vi "Add User.vi"(8 "error in":errorcluster) -> (0 "error Out":errorcluster)   [LabVIEW 2022 SP3]
uses:
  <vilib>/Utility/file.llb/Read Delimited Spreadsheet (string).vi
  <vilib>/Utility/file.llb/Write Delimited Spreadsheet (string).vi
panel:
  in  "EXIT":bool
  out "Decoded Data":string[][](array[string])
  in  "ACCESS LEVEL":string(combo)
  in  "Add User":bool
  in  "ADD-USER":string[][](array[string])
  in  "AUTH-PASS":string
  in  "AUTH-USER":string
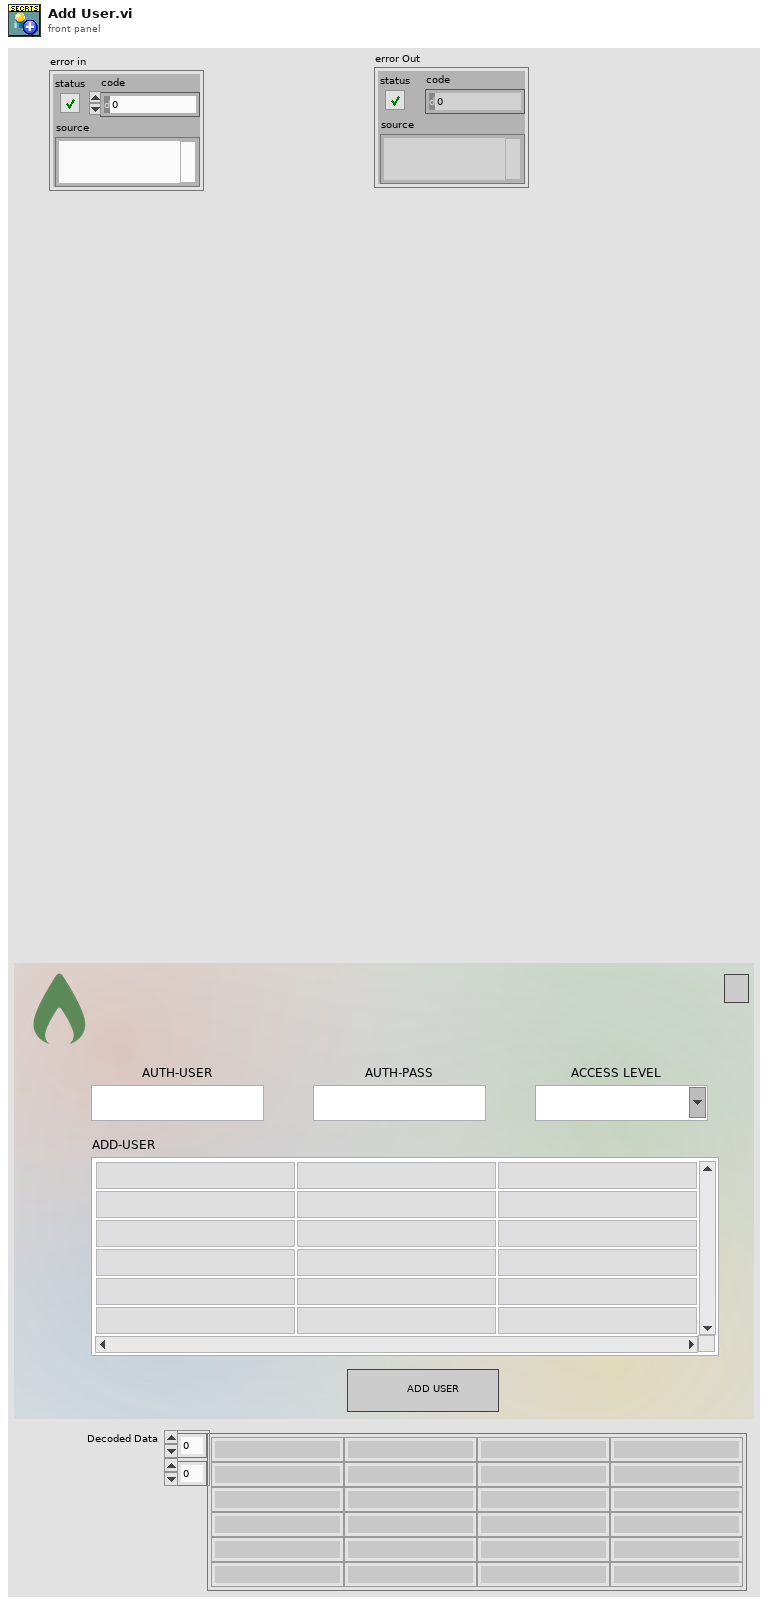
[diagram p1: front panel]
types:
  T1 = enum16{"Initialize", "Poll", "Verify User", "Wrong User", "Add User", "Exit"}
  T2 = cluster{"AUTH-USER":string, "AUTH-PASS":string, "ACCESS LEVEL":string}
  T3 = typedef "SeCrTs-file folder ctl.ctl" = cluster{"Datalog path":path, "Configuration path":path, "Signal list path":path, "Sub vi's":path, "Authentication":path, "Sequence":path, "Event Log":path, "CS Error log":path, "RT Error Log":path}
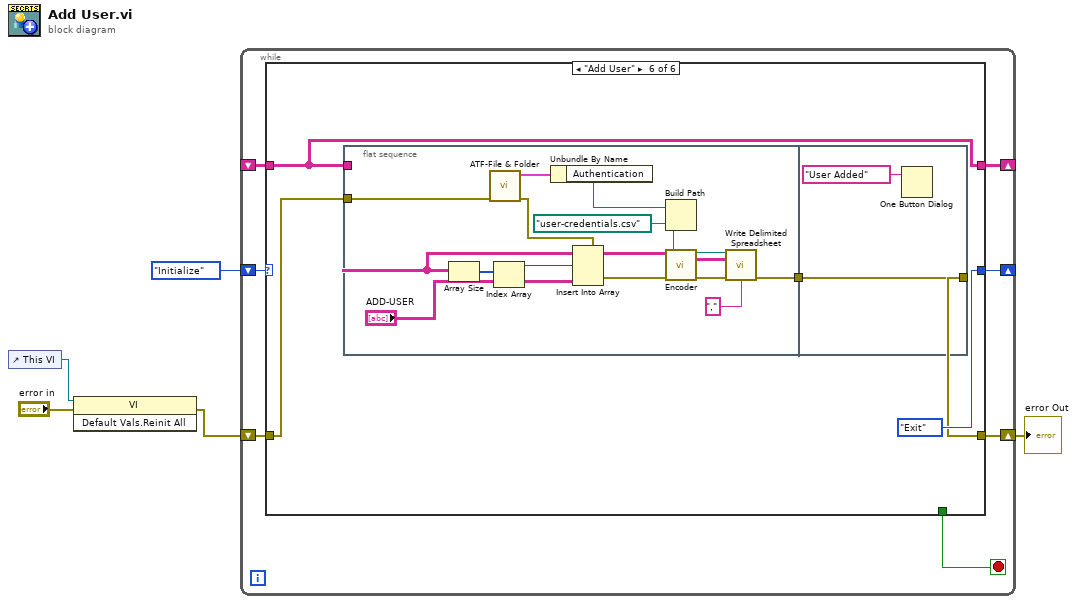
[diagram p0: block diagram]
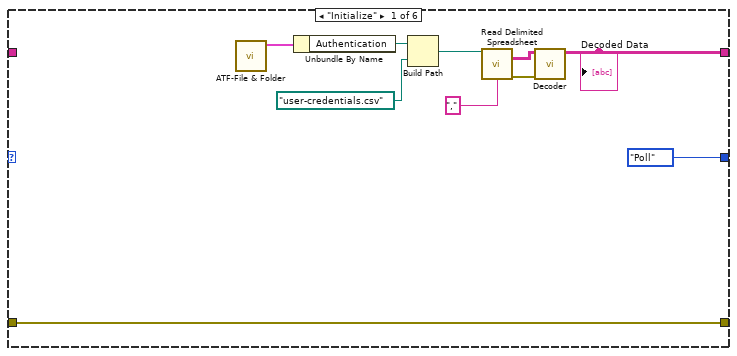
[diagram p2: hidden frame]
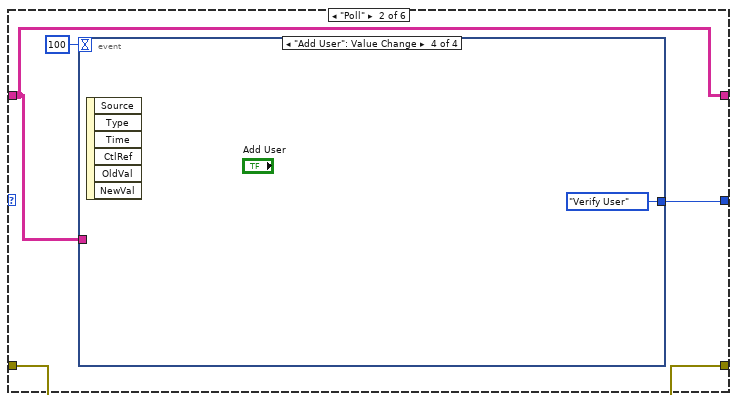
[diagram p3: hidden frame]
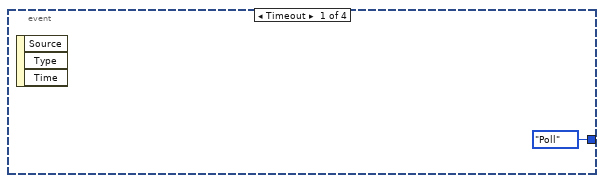
[diagram p4: hidden frame]
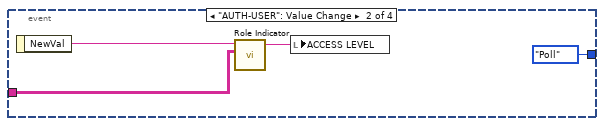
[diagram p5: hidden frame]
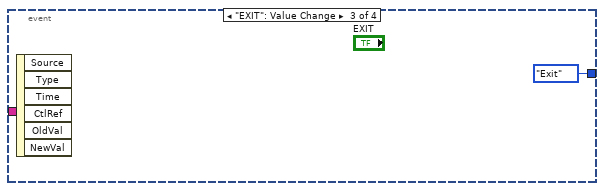
[diagram p6: hidden frame]
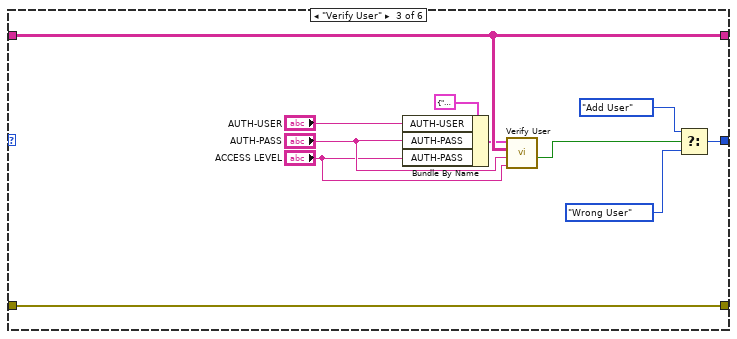
[diagram p7: hidden frame]
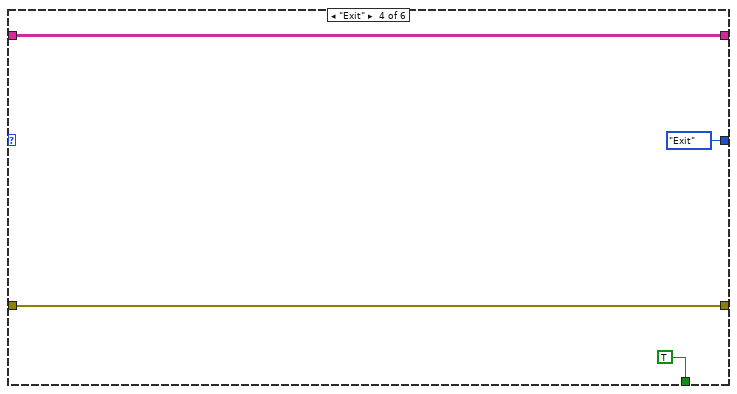
[diagram p8: hidden frame]
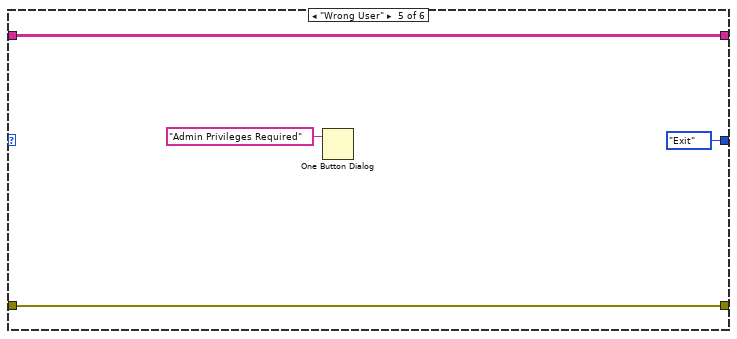
[diagram p9: hidden frame]
diagram:
  n1 = control-ref of="This VI"() -> (w3:refnum<vi>)
  n2 = invoke class="VI" method="Default Vals.Reinit All"(reference=w3, error in="error in") -> (error out=w1:errorcluster)  [unwired: 1 in, 2 out]
  n3 = while {
    shift-right: [w11] -> _
    shift-left: T1."Initialize" -> [w12]
    shift-right: [w9] -> _
    shift-left: _ -> [w8]
    shift-right: [w6] -> w4
    shift-left: w1 -> [w10]
    stop <- w7 stop-if-true
    n4 = case shown="\"Add User\"" w12 {
      tunnel: [T1."Poll" w26 w42 T1."Exit" T1."Exit" T1."Exit"] -> w11
      tunnel: w10 -> [w15 w25 w37 w45 w49 w54]
      tunnel: [w14 w23 w41 w48 w50 w56] -> w9
      tunnel: w8 -> [_ w23 w41 w48 w50 w56]
      tunnel: [_ _ _ TRUE _ _] -> w7
      tunnel: [w15 w25 w37 w45 w49 w53] -> w6
      frame "Initialize" {
        n5 = call "ATF-File & Folder.vi"() -> ("File Output"=w13:T3)  [unwired: 10 in, 1 out]
        n6 = Unbundle By Name(w13) -> ("Authentication"=w20:path)
        n7 = Build Path(base path=w20, name or relative path=path "user-credentials.csv") -> (appended path=w19:path)
        n8 = call-poly <vilib>:"Read Delimited Spreadsheet.vi"("file path (dialog if empty)"=w19, "delimiter (\\t)"="," ("delimiter (\\t)")) -> ("all rows"=w21:string[][], "error out"=w18:errorcluster)  [unwired: 8 in, 4 out]
        n9 = call "Decoder.vi"("error in"=w18, "Encoded Data"=w21) -> ("Decoded Data"=w14:string[][])  [unwired: 8 in, 1 out]
        "Decoded Data" <- w14
      }
      frame "Poll" {
        n10 = event shown="[3] \"Add User\": Value Change" {
          selector: _ -> [_ _ _ _]
          dyn-events: _ -> [_ _ _ _]
          timeout: 100 -> [_ _ _ _]
          tunnel: [T1."Poll" T1."Poll" T1."Exit" T1."Verify User"] -> w26
          tunnel: w23 -> [_ w30 _ _]
          event Timeout {
            n11 = event-data() -> ()  [unwired: 1 in, 3 out]
          }
          event "AUTH-USER": Value Change {
            n12 = event-data() -> ("NewVal"=w31:string)  [unwired: 1 in]
            n13 = call "Role Indicator.vi"("Decoded Data"=w30, "NewVal"=w31) -> ("String"=w29:string)  [unwired: 9 in]
            n14 = local write "ACCESS LEVEL"(w29) -> ()
          }
          event "EXIT": Value Change {
            n15 = event-data() -> ()  [unwired: 1 in, 6 out]
          }
          event "Add User": Value Change {
            n16 = event-data() -> ()  [unwired: 1 in, 6 out]
          }
        }
      }
      frame "Verify User" {
        n17 = Bundle By Name(cluster=T2 {"AUTH-USER"="", "AUTH-PASS"="", "ACCESS LEVEL"=""}, "AUTH-USER"="AUTH-USER", "AUTH-PASS"="AUTH-PASS", "AUTH-PASS"="ACCESS LEVEL") -> (w34:T2)
        n18 = call "Verify User.vi"("ROLE"="ACCESS LEVEL", "OLD PASSWORD in"="AUTH-PASS", "Authenticated Data"=w41, "User Cred"=w34) -> ("Administator?"=w38:bool)  [unwired: 5 in, 2 out]
        n19 = Select(t=T1."Add User", s=w38, f=T1."Wrong User") -> (s? t:f=w42:T1)
      }
      frame "Exit" {
      }
      frame "Wrong User" {
        n20 = One Button Dialog(message="Admin Privileges Required") -> ()  [unwired: 1 in, 1 out]
      }
      frame "Add User" {
        n21 = flat-sequence {
          tunnel: [w66] -> w57
          tunnel: w56 -> [w62]
          tunnel: w54 -> [w59]
          tunnel: [w74] -> w53
          tunnel: w57 -> [w74]
          frame #0 {
            n22 = Array Size(array=w62) -> (size(s)=w64:i32[])
            n23 = call "ATF-File & Folder.vi"("error in (no error)"=w59) -> ("error out"=w58:errorcluster, "File Output"=w60:T3)  [unwired: 9 in]
            n24 = Index Array(array=w64) -> (element=w65:i32)  [unwired: 1 in]
            n25 = Unbundle By Name(w60) -> ("Authentication"=w70:path)
            n26 = Insert Into Array(array=w62, index (row)=w65, new element="ADD-USER") -> (w63:string[][])  [unwired: 1 in]
            n27 = Build Path(base path=w70, name or relative path=path "user-credentials.csv") -> (appended path=w71:path)
            n28 = call "Encoder.vi"("error in"=w58, "Orginal Data"=w63) -> ("error Out"=w67:errorcluster, "Encoded Data"=w72:string[][])  [unwired: 8 in]
            n29 = call-poly <vilib>:"Write Delimited Spreadsheet.vi"("file path (dialog if empty)"=w71, "2D data"=w72, "error in (no error)"=w67, "delimiter (\\t)"="," ("delimiter (\\t)")) -> ("error out"=w66:errorcluster)  [unwired: 10 in, 1 out]
          }
          frame #1 {
            n30 = One Button Dialog(message="User Added") -> ()  [unwired: 1 in, 1 out]
          }
        }
      }
    }
  }
  "error Out" <- w4
